vi "create.AddOrderShort.vi"(11 "AddOrderShort.Parameters":T1={"Time Offset"=447000, "Order Id"="ORID0001", "Quantity"=20000, "Symbol"="AAPL", "Side Indicator"="B", "Price"=0.905}) -> (2 "Bytes.Out":u8[](array[numeric])=[34, 33, 24, 210, 6, 0, 79, 82, 73, 68, 48, 48, 48, 49, 66, 32, 78, 0, 0, 65, 65, 80, 76, 32, 32, 90, 35, 0, 0, 0, 0, 0, 0, 1] format="%.0x", 3 "MessageBase out":refnum<class "AddOrderShort.lvclass">)   [LabVIEW 2020]
uses:
  AddOrder/AddOrderShort.Parameters.ctl
  AddOrder/AddOrderShort.lvclass
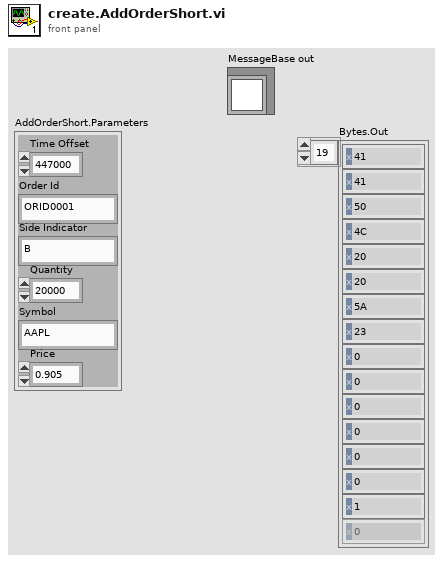
[diagram p1: front panel]
types:
  T1 = typedef "AddOrderShort.lvclass/AddOrderShort.Parameters.ctl" = cluster{"Time Offset":u32, "Order Id":string, "Quantity":u32, "Symbol":string, "Side Indicator":string, "Price":dbl}
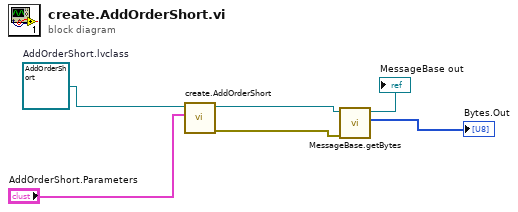
[diagram p0: block diagram]
diagram:
  w3 = refnum<class "AddOrderShort.lvclass"> refnum  # AddOrderShort.lvclass
  n1 = call-dynamic "create.AddOrderShort.vi"("AddOrderShort.Parameters"="AddOrderShort.Parameters", "AddOrderShort in"=w3) -> ("error out"=w5:errorcluster, "AddOrderShort out"=w4:refnum<class "AddOrderShort.lvclass">)  [unwired: 8 in]
  n2 = call-dynamic "MessageBase.getBytes.vi"("error in (no error)"=w5, "MessageBase in"=w4) -> ("Bytes.out"=→"Bytes.Out":u8[], "MessageBase out"=→"MessageBase out":refnum<class "AddOrderShort.lvclass">)  [unwired: 7 in, 1 out]
